vi "Create PPL.vi"(0 "Project Refnum":refnum<vi>, 5 "Build specification name":string, 11 "error in (no error)":errorcluster) -> (4 "project ref out":refnum<vi>, 6 "path":path, 15 "error out":errorcluster)   [LabVIEW 2021, in "NI_AB_API_PPL_Extensions.lvclass"]
uses:
  NI_AB_API_PPL_Extensions.lvclass
  G Plugin Editor.lvlib
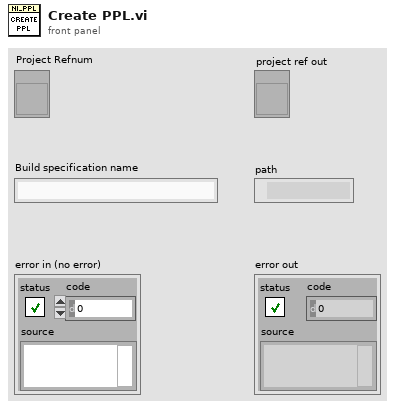
[diagram p1: front panel]
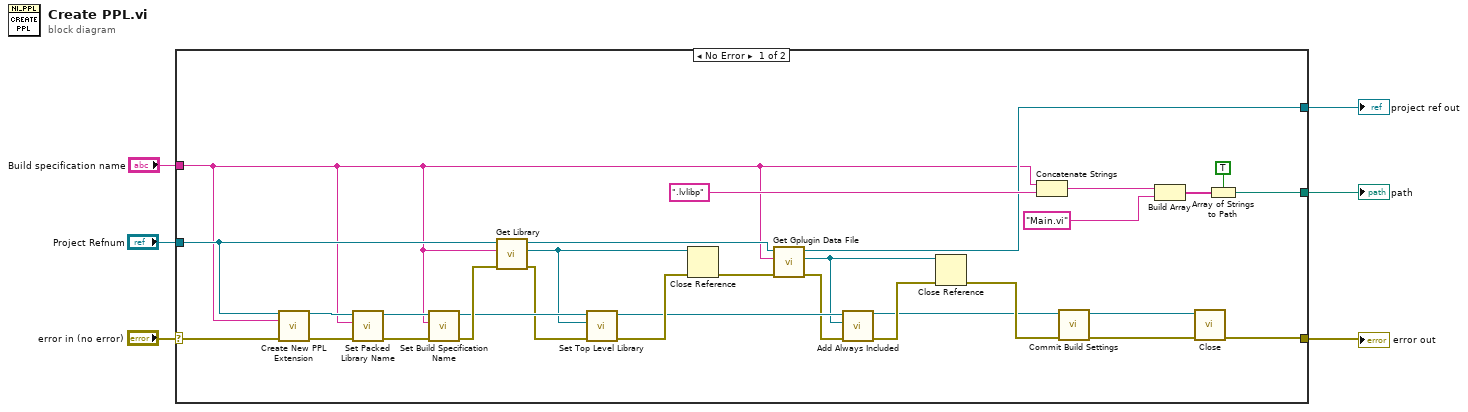
[diagram p0: block diagram]
diagram:
  n1 = case shown="No Error" "error in (no error)" {
    selector: "error in (no error)" -> [w36 w38]
    tunnel: [w24 w38] -> w6
    tunnel: "Project Refnum" -> [w35 w37]
    tunnel: "Build specification name" -> [w14 _]
    tunnel: [w15 w37] -> w2
    tunnel: [w21 _] -> w1
    frame No Error {
      n2 = call "Create New PPL Extension.vi"("Project Refnum"=w35, "Build specification name"=w14, "error in (no error)"=w36) -> ("NI_AB_API_Build out"=w20:refnum<class "NI_AB_API_PPL_Extensions.lvclass">, "error out"=w17:errorcluster)  [unwired: 11 in]
      n3 = call-dynamic "Set Packed Library Name.vi"("error in (no error)"=w17, "Packed library name"=w14, "PPL in"=w20) -> ("error out"=w18:errorcluster, "PPL out"=w19:refnum<class "NI_AB_API_PPL_Extensions.lvclass">)  [unwired: 7 in]
      n4 = call-dynamic "Set Build Specification Name.vi"("error in (no error)"=w18, "Build Specification Name"=w14, "NI_AB_API_PPL in"=w19) -> ("error out"=w34:errorcluster, "NI_AB_API_PPL out"=w33:refnum<class "NI_AB_API_PPL_Extensions.lvclass">)  [unwired: 7 in]
      n5 = call "Get Library.vi"("error in (no error)"=w34, "library name"=w14, "project ref"=w35) -> ("error out"=w32:errorcluster, "library item"=w25:refnum<vi>, "project ref out"=w16:refnum<vi>)  [unwired: 5 in, 1 out]
      n6 = call-dynamic "Set Top Level Library.vi"("error in (no error)"=w32, "ProjectItem Refnum"=w25, "PPL in"=w33) -> ("error out"=w30:errorcluster, "PPL out"=w13:refnum<class "NI_AB_API_PPL_Extensions.lvclass">)  [unwired: 7 in]
      n7 = Close Reference(reference=w25, error in (no error)=w30) -> (error out=w7:errorcluster)
      n8 = call "Get Gplugin Data File.vi"("error in (no error)"=w7, "library name"=w14, "project ref"=w16) -> ("error out"=w8:errorcluster, "Document item"=w12:refnum<vi>, "project ref out"=w15:refnum<vi>)  [unwired: 5 in, 1 out]
      n9 = call-dynamic "Add Always Included.vi"("error in (no error)"=w8, "ProjectItem Refnum"=w12, "PPL in"=w13) -> ("error out"=w11:errorcluster, "PPL out"=w9:refnum<class "NI_AB_API_PPL_Extensions.lvclass">)  [unwired: 7 in]
      n10 = Close Reference(reference=w12, error in (no error)=w11) -> (error out=w10:errorcluster)
      n11 = Concatenate Strings(w14, ".lvlibp" ("string")) -> (w27:string)
      n12 = call-dynamic "Commit Build Settings.vi"("error in (no error)"=w10, "PPL in"=w9) -> ("error out"=w31:errorcluster, "PPL out"=w26:refnum<class "NI_AB_API_PPL_Extensions.lvclass">)  [unwired: 8 in]
      n13 = Build Array(w27, "Main.vi" ("element")) -> (w22:string[])
      n14 = call-dynamic "Close.vi"("error in (no error)"=w31, "DLL in"=w26) -> ("error out"=w24:errorcluster)  [unwired: 9 in]
      n15 = Array of Strings to Path(0:w22, 1:TRUE ("relative")) -> (2:w21:path)
    }
    frame Error {
    }
  }
  "error out" <- w6
  "project ref out" <- w2
  "path" <- w1
